vi "Flywheels.vi"() -> ()   [LabVIEW 2016]
doc: "The myRIO Project template acquires acceleration data from the onboard accelerometer and displays the changes of acceleration values in a waveform chart."
uses:
  <vilib>/myRIO/Common/Instrument Driver Framework/myRIO v1.0/UART/vis/myRIO v1.0 Close UART.vi
  <vilib>/Utility/error.llb/Error Cluster From Error Code.vi
  <vilib>/myRIO/Common/Instrument Driver Framework/myRIO v1.0/PWM/vis/myRIO v1.0 Write PWM.vi
  <vilib>/myRIO/Common/Instrument Driver Framework/Utilities/vis/FPGA Ref Manager.vi
  <vilib>/myRIO/Common/Instrument Driver Framework/myRIO v1.0/myRIO v1.0 Reset FPGA.vi
  <vilib>/myRIO/Common/Instrument Driver Framework/myRIO v1.0/IRQ/vis/myRIO v1.0 IRQ Info FGV.vi
  <vilib>/myRIO/Common/Instrument Driver Framework/myRIO v1.0/IRQ/vis/myRIO v1.0 Timer IRQ Info FGV.vi
  <vilib>/myRIO/Common/Instrument Driver Framework/myRIO v1.0/IRQ/vis/myRIO v1.0 ISR Agent.vi
  <vilib>/myRIO/Instrument Drivers/Utilities/Utilities.lvlib
  <vilib>/myRIO/Instrument Drivers/Onboard IO/PWM/PWM.lvlib
panel:
  in  "Start":bool
  out "Boolean 3":bool
  out "Boolean 2":bool
  out "Boolean":bool
  out "Numeric":dbl
  in  "Duty Cycle 2":dbl min=0.0 max=0.08
  in  "Duty Cycle 1":dbl min=0.0 max=0.08
  in  "Duty Cycle 0":dbl min=0.0 max=0.08
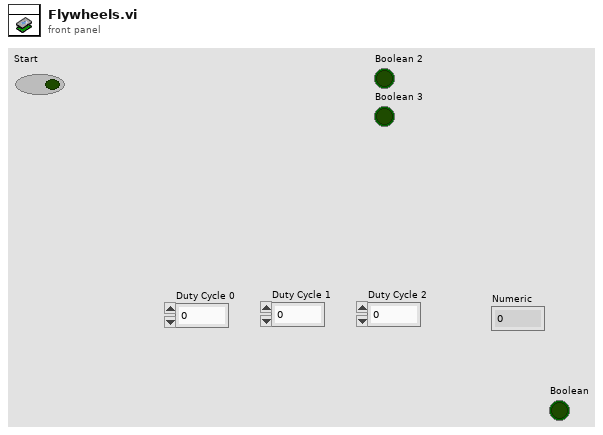
[diagram p1: front panel]
types:
  T1 = typedef "PWM.lvlib/PWM Reference.ctl" = cluster{"myRIO Reference":T2, "PWM Channels Enum":T6, "PWM Configuration":T7}
  T2 = typedef "myRIO Generic Hardware Reference.ctl" = cluster{"myRIO Model":T3, "myRIO Hardware Reference":T4}
  T3 = typedef "Hardware Version Enum.ctl" = enum16{"Unknown", "myRIO-1900", "myRIO-1950", "roboRIO", "NI ELVIS RIO CM"}
  T4 = typedef "myRIO v1.0 Reference.ctl" = cluster{"Generic FPGA Reference":T5, "Allow multiple opens":bool}
  T5 = typedef "Generic FPGA Reference.ctl" = refnum<k20>
  T6 = typedef "PWM Channels Enum.ctl" = enum16{"Not Connected", "C/PWM0", "C/PWM1", "A/PWM0", "A/PWM1", "A/PWM2", "B/PWM0", "B/PWM1", "B/PWM2", "PWM/PWM0", "PWM/PWM1", "PWM/PWM2", "PWM/PWM3", "PWM/PWM4", "PWM/PWM5", "PWM/PWM6", "PWM/PWM7", "PWM/PWM8", "PWM/PWM9"}
  T7 = typedef "PWM.lvlib/PWM Configuration.ctl" = cluster{"Frequency":dbl, "Duty Cycle":dbl}
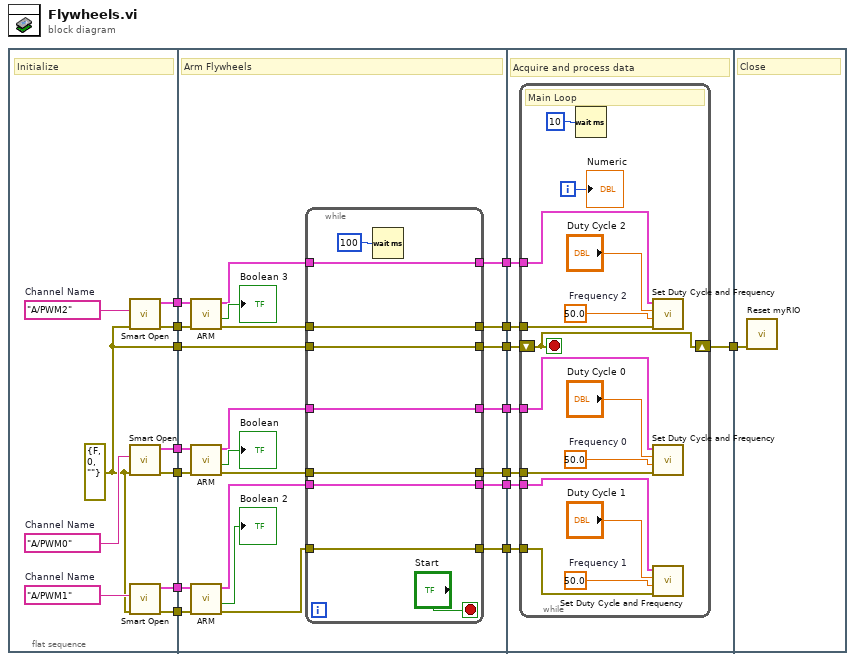
[diagram p0: block diagram]
diagram:
  n1 = flat-sequence {
    tunnel: [w20] -> w14
    tunnel: [w25] -> w13
    tunnel: [w24] -> w12
    tunnel: [w19] -> w11
    tunnel: [w18] -> w10
    tunnel: [w17] -> w9
    tunnel: [w16] -> w8
    tunnel: w14 -> [w39]
    tunnel: w13 -> [w48]
    tunnel: w12 -> [w47]
    tunnel: w11 -> [w46]
    tunnel: w10 -> [w45]
    tunnel: w9 -> [w44]
    tunnel: w8 -> [w43]
    tunnel: [w34] -> w7
    tunnel: [w32] -> w6
    tunnel: [w30] -> w5
    tunnel: [w28] -> w4
    tunnel: [w38] -> w3
    tunnel: [w36] -> w2
    tunnel: [w26] -> w1
    tunnel: [w65] -> w15
    tunnel: w7 -> [w64]
    tunnel: w6 -> [w63]
    tunnel: w5 -> [w62]
    tunnel: w4 -> [w61]
    tunnel: w3 -> [w58]
    tunnel: w2 -> [w60]
    tunnel: w1 -> [w59]
    tunnel: w15 -> [w81]
    frame #0 {
      w21 = tag "A/PWM2"  # Channel Name
      w22 = tag "A/PWM1"  # Channel Name
      w23 = tag "A/PWM0"  # Channel Name
      w20 = errorcluster {"status"=FALSE, "code"=0, "source"=""} ("error in (no error)")
      # "Initialize"
      n2 = call <vilib>:"Smart Open.vi"("error in (no error)"=w20, "Channel Name"=w21) -> ("error out"=w16:errorcluster, "PWM Ref Out"=w17:T1)  [unwired: 8 in]
      n3 = call <vilib>:"Smart Open.vi"("error in (no error)"=w20, "Channel Name"=w23) -> ("error out"=w24:errorcluster, "PWM Ref Out"=w25:T1)  [unwired: 8 in]
      n4 = call <vilib>:"Smart Open.vi"("error in (no error)"=w20, "Channel Name"=w22) -> ("error out"=w18:errorcluster, "PWM Ref Out"=w19:T1)  [unwired: 8 in]
    }
    frame #1 {
      # "Arm Flywheels"
      n5 = call "ARM.vi"("error in (no error)"=w43, "PWM Ref in"=w44) -> ("error out"=w29:errorcluster, "Boolean"=→"Boolean 3":bool, "PWM Ref out"=w31:T1)  [unwired: 7 in]
      n6 = call "ARM.vi"("error in (no error)"=w47, "PWM Ref in"=w48) -> ("error out"=w37:errorcluster, "Boolean"=→"Boolean":bool, "PWM Ref out"=w27:T1)  [unwired: 7 in]
      n7 = call "ARM.vi"("error in (no error)"=w45, "PWM Ref in"=w46) -> ("error out"=w33:errorcluster, "Boolean"=→"Boolean 2":bool, "PWM Ref out"=w35:T1)  [unwired: 7 in]
      n8 = while {
        tunnel: w39 -> [w56]
        tunnel: [w56] -> w38
        tunnel: [w55] -> w36
        tunnel: w37 -> [w55]
        tunnel: [w54] -> w34
        tunnel: w35 -> [w54]
        tunnel: [w53] -> w32
        tunnel: w33 -> [w53]
        tunnel: [w52] -> w30
        tunnel: w31 -> [w52]
        tunnel: [w51] -> w28
        tunnel: w29 -> [w51]
        tunnel: [w49] -> w26
        tunnel: w27 -> [w49]
        stop <- "Start" stop-if-true
        n9 = Wait (ms)(milliseconds to wait=u32 100) -> ()  [unwired: 1 out]
      }
    }
    frame #2 {
      # "Acquire and process data"
      n10 = while {
        shift-right: [w79] -> w65
        shift-left: w58 -> [w79]
        tunnel: w60 -> [w70]
        tunnel: w59 -> [w71]
        tunnel: w64 -> [w69]
        tunnel: w63 -> [w68]
        tunnel: w62 -> [w67]
        tunnel: w61 -> [w66]
        i -> [w78]
        stop <- w79 stop-if-true
        w76 = 50.0  # Frequency 0
        w73 = 50.0  # Frequency 2
        w75 = 50.0  # Frequency 1
        # "Main Loop"
        n11 = Wait (ms)(milliseconds to wait=u32 10) -> ()  [unwired: 1 out]
        n12 = call <vilib>:"Set Duty Cycle and Frequency.vi"("error in (no error)"=w66, "Frequency [Hz]"=w73, "Duty Cycle"="Duty Cycle 2", "PWM Ref In"=w67) -> ()  [unwired: 5 in, 2 out]
        n13 = call <vilib>:"Set Duty Cycle and Frequency.vi"("error in (no error)"=w70, "Frequency [Hz]"=w76, "Duty Cycle"="Duty Cycle 0", "PWM Ref In"=w71) -> ()  [unwired: 5 in, 2 out]
        n14 = call <vilib>:"Set Duty Cycle and Frequency.vi"("error in (no error)"=w68, "Frequency [Hz]"=w75, "Duty Cycle"="Duty Cycle 1", "PWM Ref In"=w69) -> ()  [unwired: 5 in, 2 out]
        "Numeric" <- w78
      }
    }
    frame #3 {
      # "Close"
      n15 = call <vilib>:"Reset myRIO.vi"("error in (no error)"=w81) -> ()  [unwired: 10 in, 1 out]
    }
  }
